vi "Stop Pumps (SubVI).vi"(2 "error out 2":errorcluster, 3 "VISA resource name out 2":refnum<visa-resource-name>) -> (0 "error out":errorcluster, 1 "VISA resource name out":refnum<visa-resource-name>)   [LabVIEW 2020]
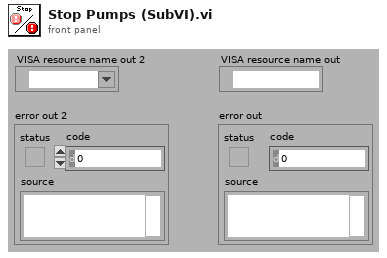
[diagram p1: front panel]
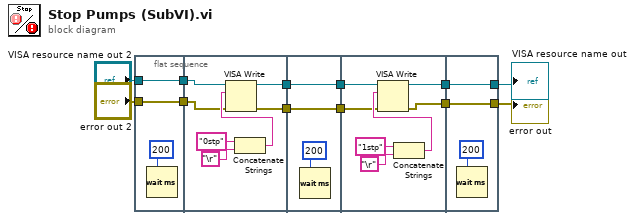
[diagram p0: block diagram]
diagram:
  n1 = flat-sequence {
    tunnel: [w14] -> w12
    tunnel: "VISA resource name out 2" -> [w14]
    tunnel: [w13] -> w11
    tunnel: "error out 2" -> [w13]
    tunnel: [w19] -> w10
    tunnel: [w18] -> w9
    tunnel: w12 -> [w16]
    tunnel: w11 -> [w17]
    tunnel: w10 -> [w24]
    tunnel: [w24] -> w8
    tunnel: [w23] -> w7
    tunnel: w9 -> [w23]
    tunnel: w8 -> [w29]
    tunnel: w7 -> [w28]
    tunnel: [w27] -> w6
    tunnel: [w26] -> w5
    tunnel: [w34] -> w4
    tunnel: w6 -> [w34]
    tunnel: [w33] -> w3
    tunnel: w5 -> [w33]
    frame #0 {
      n2 = Wait (ms)(milliseconds to wait=u32 200) -> ()  [unwired: 1 out]
    }
    frame #1 {
      n3 = Concatenate Strings("0stp" ("string"), "\r") -> (w20:string)
      n4 = VISA Write(VISA resource name=w16, write buffer=w20, error in (no error)=w17) -> (VISA resource name out=w19:refnum<visa-resource-name>, error out=w18:errorcluster)  [unwired: 1 out]
    }
    frame #2 {
      n5 = Wait (ms)(milliseconds to wait=u32 200) -> ()  [unwired: 1 out]
    }
    frame #3 {
      n6 = Concatenate Strings("1stp" ("string"), "\r") -> (w30:string)
      n7 = VISA Write(VISA resource name=w29, write buffer=w30, error in (no error)=w28) -> (VISA resource name out=w27:refnum<visa-resource-name>, error out=w26:errorcluster)  [unwired: 1 out]
    }
    frame #4 {
      n8 = Wait (ms)(milliseconds to wait=u32 200) -> ()  [unwired: 1 out]
    }
  }
  "VISA resource name out" <- w4
  "error out" <- w3
